vi "Single Engine Main.vi"() -> ()   [LabVIEW 2013]
uses:
  <vilib>/NI/Module Execution Interface/Engine Runtime/Execution States.ctl
  <vilib>/NI/Module Execution Interface/Engine Runtime/Engine Runtime Interface.lvclass
  <vilib>/NI/Tag Bus Data Framework/Framework Configuration Classes/target runtime/PL_Target Runtime.lvclass
  <vilib>/NI/Current Value Table/DataTypes/Double_Read.vi
  <vilib>/NI/Current Value Table/DataTypes/Double_Write.vi
  <vilib>/NI/Current Value Table/Type to Enum.vi
  <vilib>/NI/Current Value Table/DataTypes/Double_Type To Enum.vi
  <vilib>/NI/Current Value Table/FGVs/CVT Globals.vi
  <vilib>/NI/Current Value Table/FGVs/Tag Memory.vi
  <vilib>/NI/Current Value Table/Memory Block.vi
  <vilib>/NI/Current Value Table/DataTypes/Double_Memory Block.vi
  <vilib>/NI/Tag Bus Data Framework/Framework Configuration Classes/platypus configuration/PLConfigurationSerializer.lvlib
  <vilib>/rvi/interface/nirviOpenFPGA/nirviOpenFPGA.xnode
  <vilib>/NI/Tag Bus Module Framework/FPGA manager/FPGA manager.lvlib
  <vilib>/NI/Tag Bus Module Framework/FPGA manager/methods.ctl
  <vilib>/userdefined/High Color/nirio_resource_hc.ctl
  <vilib>/NI/Current Value Table/Current Value Table.lvlib
panel:
  in  "file path":path=path "C:/Users/Daniel/Desktop/TBDFHO/HandsOn.pcfg"
  out "C":dbl
  out "CVTReadDouble":dbl
  in  "stop CVT monitor":bool
  out "final error":errorcluster
  in  "stop":bool
  out "runtime error":errorcluster
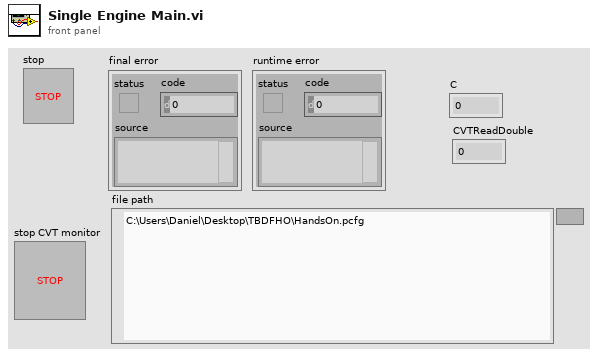
[diagram p1: front panel]
types:
  T1 = typedef "nirio_resource_hc.ctl" = tag
  T2 = typedef "FPGA manager.lvlib/methods.ctl" = enum16{"initialize bitfile", "cache bitfile", "locate bitfile", "close bitfile"}
  T3 = typedef "PLConfigurationSerializer.lvlib/file format.ctl" = cluster{"version":string, "data":string}
  T4 = typedef "PLConfigurationSerializer.lvlib/1_0_0_0 format.ctl" = cluster{"system":T5, "database":T8[]}
  T5 = typedef "PLConfigurationSerializer.lvlib/system hierarchy.ctl" = cluster{"system ID":string, "targets":T6[]}
  T6 = typedef "PLConfigurationSerializer.lvlib/target hierarchy.ctl" = cluster{"target ID":string, "engines":T7[]}
  T7 = typedef "PLConfigurationSerializer.lvlib/engine hierarchy.ctl" = cluster{"engine ID":string, "modules IDs":string[]}
  T8 = typedef "PLConfigurationSerializer.lvlib/configuration database.ctl" = cluster{"ID":string, "display name":string, "class":string, "version":string, "data":string}
  T9 = typedef "PLConfigurationSerializer.lvlib/targets cluster.ctl" = cluster{"Target Configuration":refnum<class "PL_Target Configuration.lvclass">, "engines":T10[]}
  T10 = typedef "PLConfigurationSerializer.lvlib/engines cluster.ctl" = cluster{"engine configuration":refnum<class "engine configuration.lvclass">, "modules":refnum<class "TBM module configuration.lvclass">[]}
  T11 = typedef "Engine Runtime Interface.lvclass/Execution States.ctl" = enum16{"Initializing", "Paused (Initialized)", "Running", "Set Safe Outputs", "Uninitializing", "Stopped (Uninitialized)", "Error (Uninitialized)", "Safe State (Uninitialized)", "Closed"}
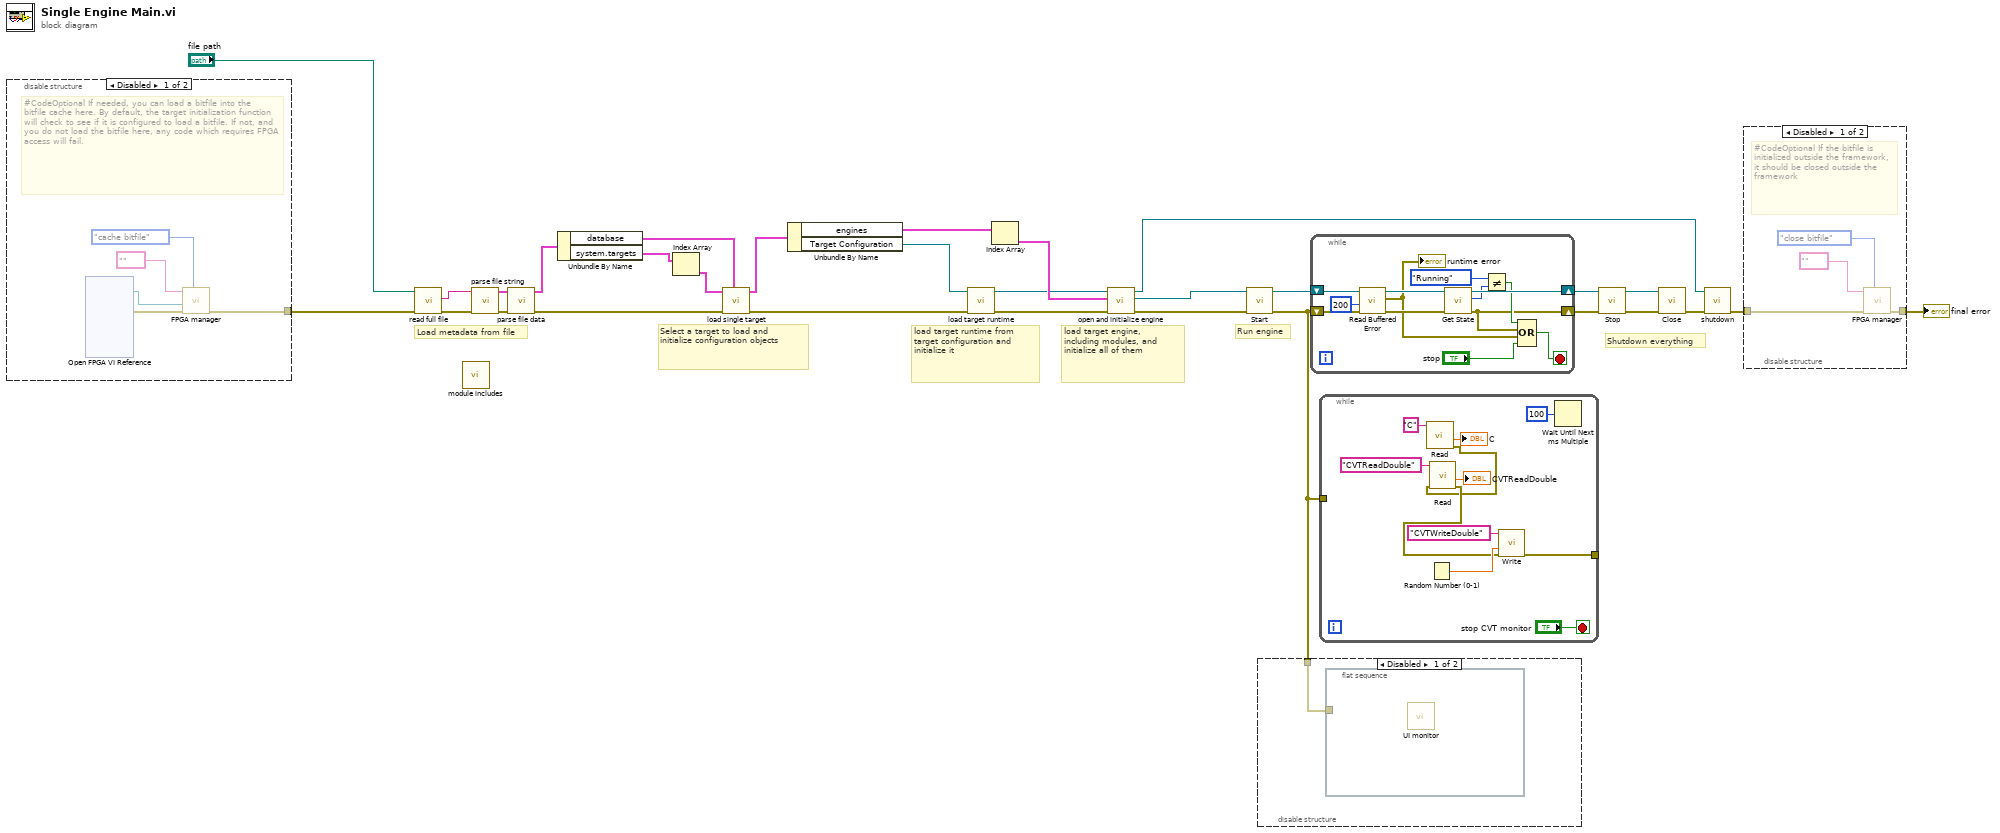
[diagram p0: block diagram]
diagram:
  # "Shutdown everything"
  # "Run engine"
  # "load target engine, including modules, and initialize all of them"
  # "load target runtime from target configuration and initialize it"
  # "Select a target to load and initialize configuration objects"
  # "Load metadata from file"
  n1 = disable-structure shown="Disabled" {
    disable-tunnel: [w31 _] -> w4
    frame Disabled {
      # "#CodeOptional If needed, you can load a bitfile into the bitfile cache here. By default, the target initialization function will check to see if it is configured to load a bitfile. If not, and you do not load the bitfile here, any code which requires FPGA access will fail."
      n2 = xnode "Open FPGA VI Reference"() -> ("FPGA VI Reference Out"=w34:refnum<k20>, "error out"=w35:errorcluster)  [unwired: 2 in]
      n3 = call <vilib>:"FPGA manager.vi"("action"=methods."cache bitfile", "error in"=w35, "bitfile to cache"=w34, "RIO resource"=T1 "") -> ("error out"=w31:errorcluster)  [unwired: 5 in, 2 out]
    }
    frame Enabled {
    }
  }
  n4 = call <vilib>:"read full file.vi"("error in"=w4, "file path"="file path") -> ("error out"=w21:errorcluster, "data"=w22:string)  [unwired: 8 in]
  n5 = call "module includes.vi"() -> ()  [unwired: 12 in]
  n6 = call <vilib>:"parse file string.vi"("error in"=w21, "data string"=w22) -> ("error out"=w23:errorcluster, "file format"=w24:T3)  [unwired: 8 in]
  n7 = call <vilib>:"parse file data.vi"("error in"=w23, "file format"=w24) -> ("error out"=w19:errorcluster, "file information"=w20:T4)  [unwired: 8 in]
  n8 = Unbundle By Name(w20) -> ("database"=w18:T8[], "system.targets"=w17:T6[])
  n9 = Index Array(array=w17) -> (element=w16:T6)  [unwired: 1 in]
  n10 = call <vilib>:"load single target.vi"("database in"=w18, "error in"=w19, "target to load"=w16) -> ("error out"=w7:errorcluster, "targets cluster out"=w15:T9)  [unwired: 7 in]
  n11 = Unbundle By Name(w15) -> ("engines"=w14:T10[], "Target Configuration"=w8:refnum<class "PL_Target Configuration.lvclass">)
  n12 = call <vilib>:"load target runtime.vi"("error in"=w7, "target configuration"=w8) -> ("error out"=w6:errorcluster, "target runtime"=w5:refnum<class "PL_Target Runtime.lvclass">)  [unwired: 8 in]
  n13 = Index Array(array=w14) -> (element=w9:T10)  [unwired: 1 in]
  n14 = call <vilib>:"open and initialize engine.vi"("error in"=w6, "engine configuration in"=w9, "Target Runtime in"=w5) -> ("error out"=w13:errorcluster, "Engine Runtime Interface out"=w12:refnum<class "Engine Runtime Interface.lvclass">, "Target Runtime out"=w10:refnum<class "PL_Target Runtime.lvclass">)  [unwired: 6 in]
  n15 = call-dynamic "Start.vi"("error in"=w13, "Engine Runtime Interface in"=w12) -> ("error out"=w1:errorcluster, "Engine Runtime Interface out"=w27:refnum<class "Engine Runtime Interface.lvclass">)  [unwired: 8 in]
  n16 = disable-structure shown="Disabled" {
    disable-tunnel: w1 -> [w36 _]
    frame Disabled {
      n17 = flat-sequence {
        tunnel: w36 -> [_]
        frame #0 {
          n18 = call "UI monitor.vi"() -> ()  [unwired: 12 in]
        }
      }
    }
    frame Enabled {
    }
  }
  n19 = while {
    shift-right: [w45] -> w26
    shift-left: w27 -> [w49]
    shift-right: [w38] -> w25
    shift-left: w1 -> [w48]
    stop <- w43 stop-if-true
    n20 = call-dynamic "Read Buffered Error.vi"("error in"=w48, "timeout in ms (0)"=200, "Engine Runtime Interface in"=w49) -> ("error out"=w46:errorcluster, "Engine Error"=w42:errorcluster, "Engine Runtime Interface out"=w47:refnum<class "Engine Runtime Interface.lvclass">)  [unwired: 6 in]
    "runtime error" <- w42
    n21 = call-dynamic "Get State.vi"("error in"=w46, "Engine Runtime Interface in"=w47) -> ("error out"=w38:errorcluster, "Engine State"=w41:T11, "Engine Runtime Interface out"=w45:refnum<class "Engine Runtime Interface.lvclass">)  [unwired: 7 in]
    n22 = Not Equal?(x=Execution_States."Running" ("Engine State"), y=w41) -> (x != y?=w39:bool)
    n23 = Compound Arithmetic op=OR(w39, w38, w42, "stop") -> (w43:bool)
  }
  n24 = while {
    tunnel: w1 -> [_]
    tunnel: [w53] -> _
    stop <- "stop CVT monitor" stop-if-true
    n25 = call-poly <vilib>:"Read.vi"("Tag Name"="C") -> ("error out"=w50:errorcluster, "Value"=→"C":dbl)  [unwired: 9 in]
    n26 = Random Number (0-1)() -> (number: 0 to 1=w56:dbl)
    n27 = call-poly <vilib>:"Read.vi"("error in (no error)"=w50, "Tag Name"="CVTReadDouble") -> ("error out"=w54:errorcluster, "Value"=→"CVTReadDouble":dbl)  [unwired: 8 in]
    n28 = call-poly <vilib>:"Write.vi"("error in (no error)"=w54, "Value"=w56, "Tag Name"="CVTWriteDouble") -> ("error out"=w53:errorcluster)  [unwired: 8 in]
    n29 = Wait Until Next ms Multiple(millisecond multiple=u32 100) -> ()  [unwired: 1 out]
  }
  n30 = call-dynamic "Stop.vi"("error in"=w25, "Engine Runtime Interface in"=w26) -> ("error out"=w28:errorcluster, "Engine Runtime Interface out"=w29:refnum<class "Engine Runtime Interface.lvclass">)  [unwired: 8 in]
  n31 = call-dynamic "Close.vi"("error in"=w28, "Engine Runtime Interface in"=w29) -> ("error out"=w11:errorcluster)  [unwired: 9 in]
  n32 = call-dynamic "shutdown.vi"("error in"=w11, "Target Runtime in"=w10) -> ("error out"=w3:errorcluster)  [unwired: 9 in]
  n33 = disable-structure shown="Disabled" {
    disable-tunnel: w3 -> [w62 w65]
    disable-tunnel: [w61 w65] -> w2
    frame Disabled {
      # "#CodeOptional If the bitfile is initialized outside the framework, it should be closed outside the framework"
      n34 = call <vilib>:"FPGA manager.vi"("action"=methods."close bitfile", "error in"=w62, "RIO resource"=T1 "") -> ("error out"=w61:errorcluster)  [unwired: 6 in, 2 out]
    }
    frame Enabled {
    }
  }
  "final error" <- w2
